vi "Find Context.vi"(11 "Name":string="Main Application Instance") -> (2 "Found?":bool, 3 "App":refnum<vi>)   [LabVIEW 2022 SP3, in "FlexBlocks Support.lvlib"]
uses:
  FlexBlocks Support.lvlib
panel:
  out "All Names":string[](array[string])
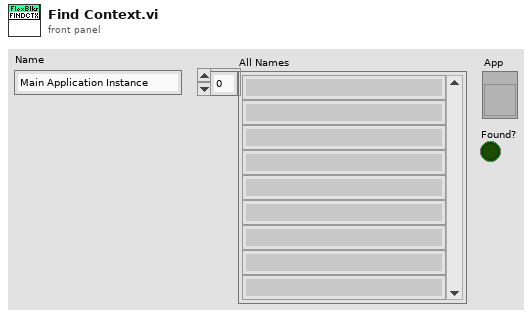
[diagram p1: front panel]
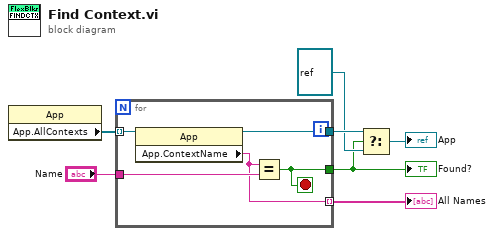
[diagram p0: block diagram]
diagram:
  n1 = property class="App"() -> ("App.AllContexts"=w7:refnum<vi>[])  [unwired: 2 in, 2 out]
  n2 = for {
    tunnel: w7 -> [w12] mode=indexing
    tunnel: "Name" -> [w11]
    tunnel: [w10] -> w5
    tunnel: [w9] -> w3
    tunnel: [w8] -> w1 mode=indexing
    stop <- w9 stop-if-true
    n3 = property class="App"(reference=w12) -> (reference out=w10:refnum<vi>, "App.ContextName"=w8:string)  [unwired: 1 in, 1 out]
    n4 = Equal?(x=w8, y=w11) -> (x = y?=w9:bool)
  }
  "Found?" <- w3
  "All Names" <- w1
  n5 = Select(t=w5, s=w3, f=refnum<vi> refnum) -> (s? t:f=→"App":refnum<vi>)
